vi "initializemotors.vi"(8 "Motor serial numbers":i32[](array[numeric]), 9 "MG17Motor Z":refnum<k7>(container), 10 "MG17Motor Y":refnum<k7>(container), 11 "MG17 Motor X":refnum<k7>(container)) -> (2 "Output errors":errorcluster[](array[cluster]), 3 "Output references":refnum<k7>[](array[refnum]))   [LabVIEW 2014]
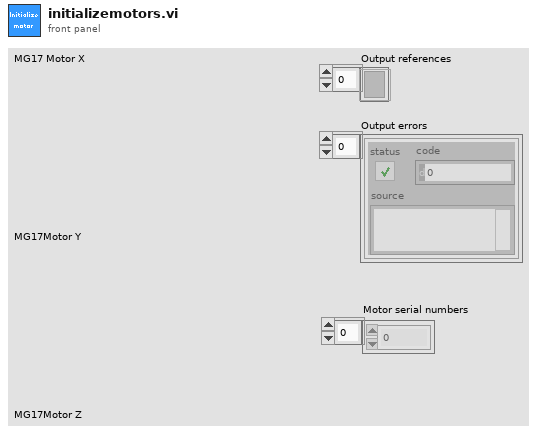
[diagram p1: front panel]
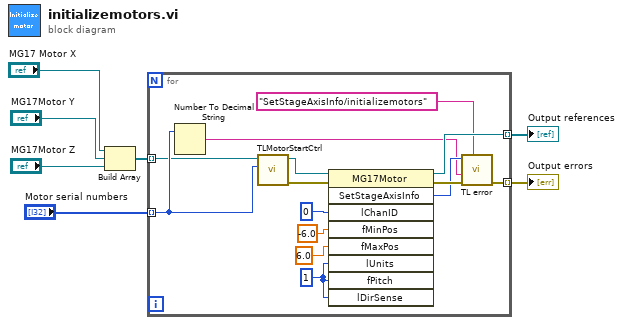
[diagram p0: block diagram]
diagram:
  n1 = Build Array("MG17 Motor X", "MG17Motor Y", "MG17Motor Z") -> (w1:refnum<k7>[])
  n2 = for {
    tunnel: [w15] -> w7 mode=indexing
    tunnel: [w17] -> w6 mode=indexing
    tunnel: "Motor serial numbers" -> [w11] mode=indexing
    tunnel: w1 -> [w10] mode=indexing
    w18 = 1 ("lUnits")
    n3 = Number To Decimal String(number=w11) -> (decimal integer string=w13:string)  [unwired: 1 in]
    n4 = call "TLMotorStartCtrl.vi"("SerialNum"=w11, "Motor Ref"=w10) -> ("Error Out"=w9:errorcluster, "Motor Ref"=w8:refnum<k7>)  [unwired: 4 in]
    n5 = invoke class="MG17Motor" method="SetStageAxisInfo"(reference=w8, error in=w9, "lChanID"=0, "fMinPos"=sgl -6.0, "fMaxPos"=sgl 6.0, "lUnits"=w18, "fPitch"=w18, "lDirSense"=w18) -> (reference out=w17:refnum<k7>, error out=w16:errorcluster, "SetStageAxisInfo"=w14:i32)  [unwired: 1 in, 6 out]
    n6 = call "TL error.vi"("Input string"="SetStageAxisInfo/initializemotors", "error in (no error)"=w16, "Serial number of motor"=w13, "Return Code"=w14) -> ("error out"=w15:errorcluster)  [unwired: 7 in]
  }
  "Output errors" <- w7
  "Output references" <- w6
